vi "Configure DC Voltage.vi"(4 "Fast Conversion (T: ON)":bool=TRUE, 6 "Filter (F: OFF)":bool, 8 "error in (no error)":errorcluster, 9 "Connection (0: Two wire)":u16(ring) items=["Two wire", "Four wire"], 11 "VISA resource name":refnum<visa-resource-name>) -> (0 "error out":errorcluster, 3 "VISA resource name out":refnum<visa-resource-name>)   [LabVIEW 2011, in "Fluke 8508.lvlib"]
doc: "This VI sets DC Voltage specific settings such as the connection, filtering and conversion type on the instrument.\n\nNOTE: .This VI does not have to run just to set the instrument to make DC voltage measuremnts, but instead it is meant to be a supplement to the \"Configure Measurement\" VI which sets the measurement function, range, and resolution."
uses:
  Fluke 8508.lvlib
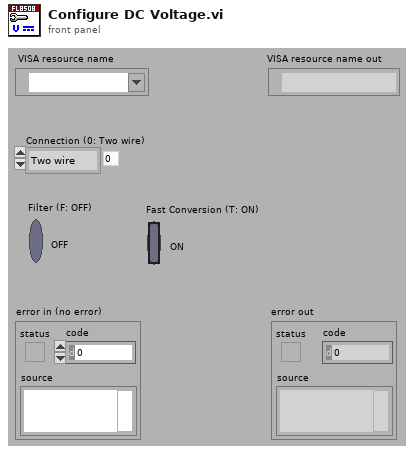
[diagram p1: front panel]
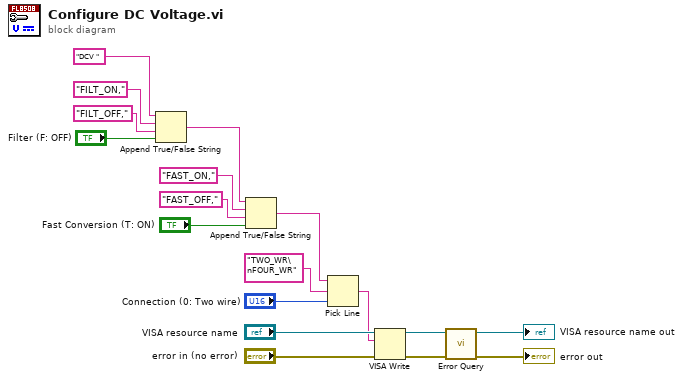
[diagram p0: block diagram]
diagram:
  n1 = Append True/False String(1:"Filter (F: OFF)", 2:"FILT_OFF," ("false string"), 3:"FILT_ON," ("true string"), 4:"DCV ") -> (0:w6:string)
  n2 = Append True/False String(1:"Fast Conversion (T: ON)", 2:"FAST_OFF," ("false string"), 3:"FAST_ON," ("true string"), 4:w6) -> (0:w9:string)
  n3 = Pick Line(string ("")=w9, multi-line string="TWO_WR\nFOUR_WR" ("true string"), line index="Connection (0: Two wire)") -> (output string=w10:string)
  n4 = VISA Write(VISA resource name="VISA resource name", write buffer=w10, error in (no error)="error in (no error)") -> (VISA resource name out=w4:refnum<visa-resource-name>, error out=w3:errorcluster)  [unwired: 1 out]
  n5 = call "Error Query.vi"("error in (no error)"=w3, "VISA resource name"=w4) -> ("error out"=→"error out":errorcluster, "VISA resource name out"=→"VISA resource name out":refnum<visa-resource-name>)  [unwired: 6 in, 2 out]
